vi "Write DAC Voltage - Multiple DUTs.vi"(0 "Channel (0-5)":u32, 5 "Voltage":dbl format="%.3f V", 7 "Vref (-1: Unchanged)":dbl=-1.0 format="%.3f V", 9 "Dev Mask (All)":bool[](array[boolean])=[TRUE, TRUE, TRUE, TRUE, TRUE, TRUE], 11 "error in":errorcluster, 12 "Log (T)":bool=TRUE, 13 "DUT (Modulo 4)":T2, 14 "FPGA":T1) -> (4 "Data Out":string, 15 "error out":errorcluster)   [LabVIEW 2017, in "Host SRL.lvlib"]
uses:
  Host SRL.lvlib
  Type Defs/WSVCAP SHL DUT Number Enum.ctl
  Type Defs/WSVCAP SHL FPGA Enum.ctl
  Type Defs/Cap and DAC Table Manager Operation Enum.ctl
panel:
  # "With all 6 devices selected in the Device Map:\n\nThis VI will write to 1 Channel, 1 DUT on Each Device (6 DUTs Total)\n\nFor example, a DUT value of any of the following: 1,5,9,13,17,21\nAll of them will be written to"
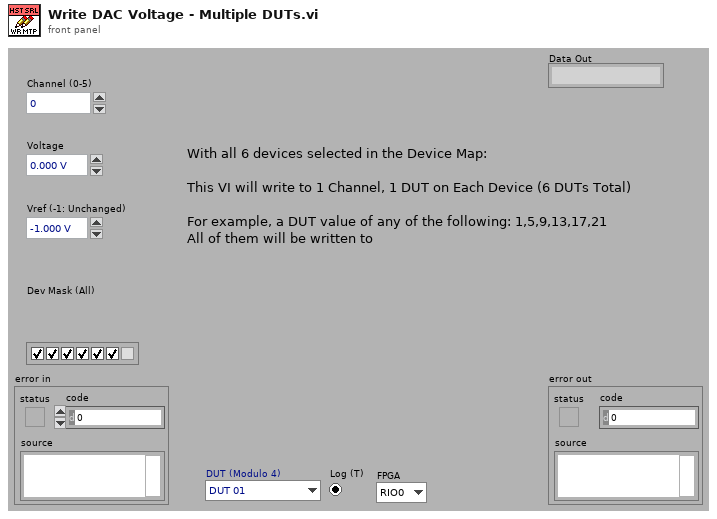
[diagram p1: front panel]
types:
  T1 = typedef "WSVCAP SHL FPGA Enum.ctl" = enum16{"RIO0", "RIO1"}
  T2 = typedef "WSVCAP SHL DUT Number Enum.ctl" = enum16{"DUT 01", "DUT 02", "DUT 03", "DUT 04", "DUT 05", "DUT 06", "DUT 07", "DUT 08", "DUT 09", "DUT 10", "DUT 11", "DUT 12", "DUT 13", "DUT 14", "DUT 15", "DUT 16", "DUT 17", "DUT 18", "DUT 19", "DUT 20", "DUT 21", "DUT 22", "DUT 23", "DUT 24"}
  T3 = typedef "Cap and DAC Table Manager Operation Enum.ctl" = enum16{"Initialize", "Add Single DAC", "Add All DAC", "Add All DUT Single DAC", "Add All Cap", "Get Status"}
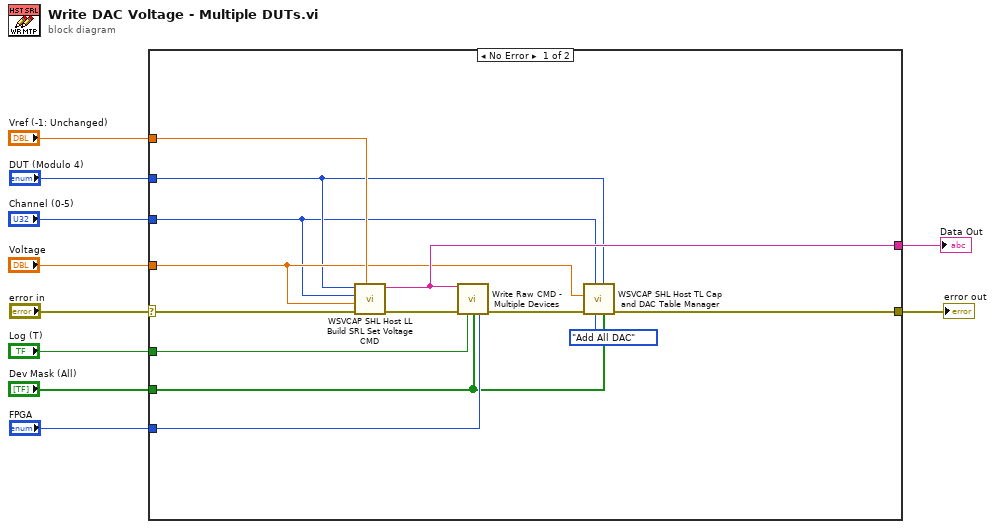
[diagram p0: block diagram]
diagram:
  n1 = case shown="No Error" "error in" {
    selector: "error in" -> [w20 _]
    tunnel: [w16 _] -> w10
    tunnel: "DUT (Modulo 4)" -> [w14 _]
    tunnel: "Log (T)" -> [w21 _]
    tunnel: "FPGA" -> [w22 _]
    tunnel: [w23 _] -> w5
    tunnel: "Channel (0-5)" -> [w13 _]
    tunnel: "Voltage" -> [w15 _]
    tunnel: "Vref (-1: Unchanged)" -> [w18 _]
    tunnel: "Dev Mask (All)" -> [w11 _]
    frame No Error {
      n2 = call "WSVCAP SHL Host LL Build SRL Set Voltage CMD.vi"("Vref (-1: Unchanged)"=w18, "error in (no error)"=w20, "Voltage (-1: Use Data Out)"=w15, "Channel (0-5)"=w13, "DUT"=w14) -> ("error out"=w19:errorcluster, "Raw CMD [Str]"=w23:string)  [unwired: 2 in, 3 out]
      n3 = call "Write Raw CMD - Multiple Devices.vi"("Data Out"=w23, "error in"=w19, "Log (T)"=w21, "Dev Mask (All)"=w11, "FPGA"=w22) -> ("error out"=w17:errorcluster)  [unwired: 10 in]
      n4 = call "WSVCAP SHL Host TL Cap and DAC Table Manager.vi"("Dev Mask (Add All DAC Only)"=w11, "DUT"=w14, "Operation"=Cap_and_DAC_Table_Manager_Operation_Enum."Add All DAC", "Channel (0-5)"=w13, "Error In"=w17, "Voltage"=w15) -> ("Error Out"=w16:errorcluster)  [unwired: 4 in, 1 out]
    }
    frame Error {
    }
  }
  "error out" <- w10
  "Data Out" <- w5
